vi "Save setup in Local PC.vi"(0 "VISA resource name":refnum<visa-resource-name>, 5 "Image File Name or Path (in scope)":path=path "C:/Users/Public/Cap_Rise.set", 7 "Path of Image in Local PC (Destination)":path, 11 "error in":errorcluster) -> (4 "VISA resource name out":refnum<visa-resource-name>, 15 "error out":errorcluster)   [LabVIEW 2019]
doc: "This VI saves the screen capture in the local PC"
uses:
  <userlib>/_TI-LA/Instr Drivers/Oscilloscope/MSO5X/Driver/MSO5X.lvlib
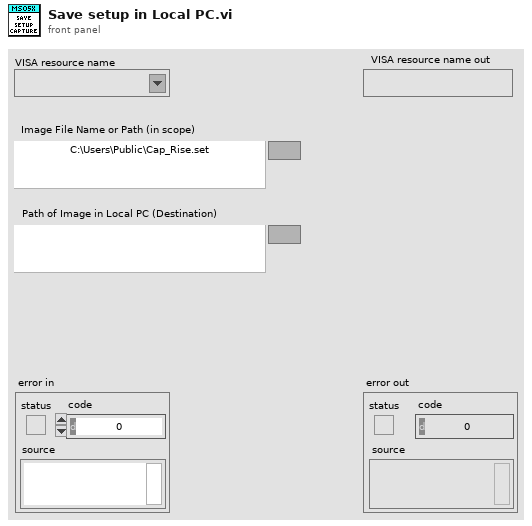
[diagram p1: front panel]
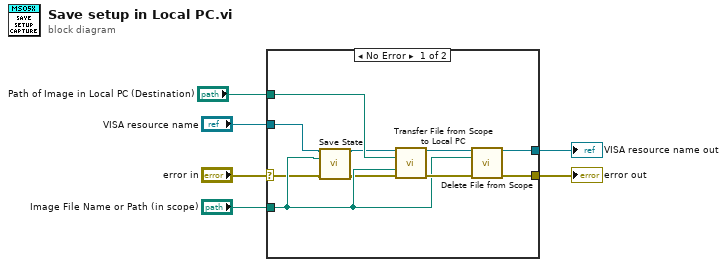
[diagram p0: block diagram]
diagram:
  n1 = case shown="No Error" "error in" {
    selector: "error in" -> [w9 w18]
    tunnel: [w15 w18] -> w5
    tunnel: "VISA resource name" -> [w11 w17]
    tunnel: "Path of Image in Local PC (Destination)" -> [w12 _]
    tunnel: "Image File Name or Path (in scope)" -> [w10 _]
    tunnel: [w16 w17] -> w1
    frame No Error {
      n2 = call <userlib>:"Save State.vi"("VISA resource name"=w11, "File Path in PC (“C:\\File.set”)"=w10, "error in"=w9) -> ("VISA resource name out"=w7:refnum<visa-resource-name>, "error out"=w8:errorcluster)  [unwired: 11 in]
      n3 = call <userlib>:"Transfer File from Scope to Local PC.vi"("VISA resource name"=w7, "Path of Image in Local PC (Destination)"=w12, "Image File Name or Path in Scope (Source)"=w10, "error in (no error)"=w8) -> ("VISA resource name out"=w13:refnum<visa-resource-name>, "error out"=w14:errorcluster)  [unwired: 10 in]
      n4 = call <userlib>:"Delete File from Scope.vi"("VISA resource name"=w13, "File Path/Directory to be deleted"=w10, "error in (no error)"=w14) -> ("VISA resource name out"=w16:refnum<visa-resource-name>, "error out"=w15:errorcluster)  [unwired: 11 in]
    }
    frame Error {
    }
  }
  "VISA resource name out" <- w1
  "error out" <- w5
